vi "2 Round Buoy.vi"() -> ()   [LabVIEW 2011]
uses:
  2 Typedefs/UTM Location.ctl
  2 Typedefs/Velocity.ctl
  2 Classes/Mission/Mission.lvclass
  2 Globals/2 Global.vi
  2 Classes/MissionQueue/MissionQueue.lvclass
  2 Classes/Waypoint/Waypoint.lvclass
panel:
  in  "Tolerance":dbl=0.5
  out "First Waypoint":T1 {"North" format="%#_10f"; "East" format="%#_8f"}
  out "Third Waypoint":T1 {"North" format="%#_10f"; "East" format="%#_8f"}
  out "Second Waypoint":T1 {"North" format="%#_10f"; "East" format="%#_8f"}
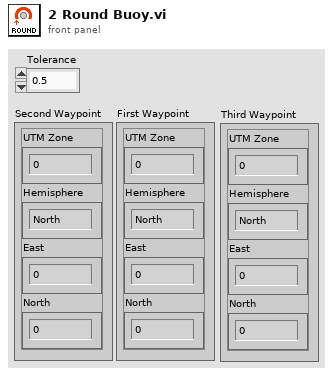
[diagram p1: front panel]
types:
  T1 = typedef "UTM Location.ctl" = cluster{"UTM Zone":dbl, "Hemisphere":enum16{"North", "South"}, "East":dbl, "North":dbl}
  T2 = typedef "Velocity.ctl" = cluster{"East":dbl, "North":dbl}
  T3 = cluster{"UTM Zone":dbl, "Hemisphere":u16, "East":dbl, "North":dbl}
  T4 = typedef "heading.ctl" = dbl
  T5 = typedef "Waypoints List.ctl" = refnum<class "Waypoint.lvclass">[]
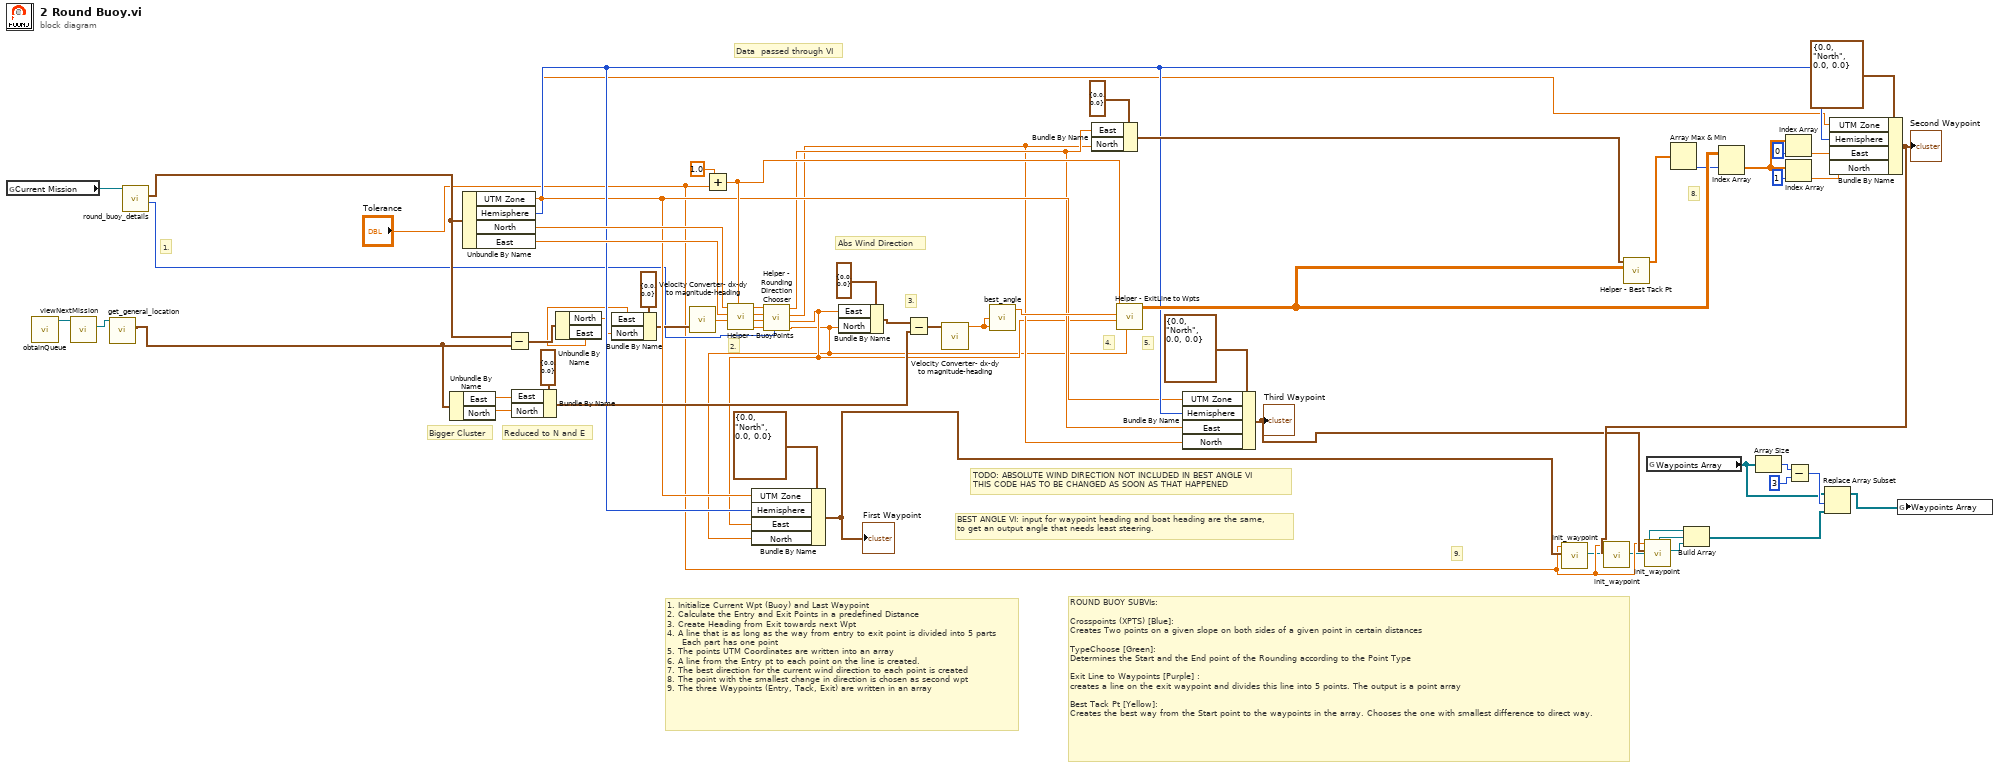
[diagram p0: block diagram]
diagram:
  # "ROUND BUOY SUBVIs:\n\nCrosspoints (XPTS) [Blue]:\nCreates Two points on a given slope on both sides of a given point in certain distances\n\nTypeChoose [Green]:\nDetermines the Start and the End point of the Rounding according to the Point Type\n\nExit Line to Waypoints [Purple] :\ncreates a line on the exit waypoint and divides this line into 5 points. The output is a point array\n\nBest Tack Pt [Yellow]:\nCreates the best way from the Start point to the waypoints in the array. Chooses the one with smallest difference to direct way."
  # "BEST ANGLE VI: input for waypoint heading and boat heading are the same,\nto get an output angle that needs least steering."
  # "Reduced to N and E"
  # "Bigger Cluster"
  # "Data  passed through VI"
  # "9."
  # "TODO: ABSOLUTE WIND DIRECTION NOT INCLUDED IN BEST ANGLE VI\nTHIS CODE HAS TO BE CHANGED AS SOON AS THAT HAPPENED"
  # "8."
  # "5."
  # "1. Initialize Current Wpt (Buoy) and Last Waypoint\n2. Calculate the Entry and Exit Points in a predefined Distance\n3. Create Heading from Exit towards next Wpt\n4. A line that is as long as the way from entry to exit point is divided into 5 parts\n     Each part has one point\n5. The points UTM Coordinates are written into an array\n6. A line from the Entry pt to each point on the line is created.\n7. The best direction for the current wind direction to each point is created\n8. The point with the smallest change in direction is chosen as second wpt\n9. The three Waypoints (Entry, Tack, Exit) are written in an array"
  # "4."
  # "3."
  # "Abs Wind Direction"
  # "2."
  # "1."
  n1 = global read "2 Global.vi" "Current Mission"() -> (w20:refnum<class "Mission.lvclass">)
  n2 = call "obtainQueue.vi"() -> ("MissionQueue.lvclass"=w17:refnum<class "MissionQueue.lvclass">)  [unwired: 10 in, 1 out]
  n3 = call "viewNextMission.vi"("MissionQueue in"=w17) -> ("Mission.lvclass"=w1:refnum<class "Mission.lvclass">)  [unwired: 7 in, 3 out]
  n4 = call "get_general_location.vi"("Mission in"=w1) -> ("General Location"=w2:T1)  [unwired: 8 in, 2 out]
  n5 = call-dynamic "round_buoy_details.vi"("Mission in"=w20) -> ("Round side?"=w18:enum16{"Starboard", "Port"}, "Buoy to Round"=w19:T1)  [unwired: 7 in, 2 out]
  n6 = Unbundle By Name(w2) -> ("East"=w58:dbl, "North"=w57:dbl)
  n7 = Unbundle By Name(w19) -> ("UTM Zone"=w35:dbl, "Hemisphere"=w36:enum16{"North", "South"}, "North"=w61:dbl, "East"=w60:dbl)
  n8 = Subtract(x=w19, y=w2) -> (x-y=w25:T3)
  n9 = Bundle By Name(cluster=T2 {"East"=0.0, "North"=0.0} ("Vector In"), "East"=w58, "North"=w57) -> (w54:T2)
  n10 = Unbundle By Name(w25) -> ("North"=w23:dbl, "East"=w16:dbl)
  n11 = Bundle By Name(cluster=T2 {"East"=0.0, "North"=0.0} ("Vector In"), "East"=w16, "North"=w23) -> (w22:T2)
  n12 = call "Velocity Converter- dx-dy to magnitude-heading.vi"("Vector In"=w22) -> ("Heading Out"=w21:T4)  [unwired: 9 in, 1 out]
  n13 = Add(x=1.0, y="Tolerance") -> (x+y=w52:dbl)
  n14 = call "Helper - BuoyPoints.vi"("Distance"=w52, "K"=w21, "East"=w60, "North"=w61) -> ("NorthOut 2"=w30:dbl, "East Out 2"=w31:dbl, "NorthOut"=w32:dbl, "East Out"=w33:dbl)  [unwired: 4 in]
  n15 = call "Helper - Rounding Direction Chooser.vi"("Enum"=w18, "Point NORTH 2"=w30, "Point EAST 2"=w31, "Point NORTH"=w32, "Point EAST"=w33) -> ("End Point NORTH"=w26:dbl, "End Point EAST"=w27:dbl, "Start Point NORTH"=w28:dbl, "Start Point EAST"=w29:dbl)  [unwired: 3 in]
  n16 = Bundle By Name(cluster=T1 {"UTM Zone"=0.0, "Hemisphere"=enum."North", "East"=0.0, "North"=0.0} ("UTM Location"), "UTM Zone"=w35, "Hemisphere"=w36, "East"=w27, "North"=w26) -> (w15:T1)
  "First Waypoint" <- w15
  n17 = Bundle By Name(cluster=T2 {"East"=0.0, "North"=0.0} ("Vector In"), "East"=w27, "North"=w26) -> (w40:T2)
  n18 = Subtract(x=w40, y=w54) -> (x-y=w53:T2)
  n19 = call "Velocity Converter- dx-dy to magnitude-heading.vi"("Vector In"=w53) -> ("Heading Out"=w34:T4)  [unwired: 9 in, 1 out]
  n20 = call "best_angle.vi"("Waypoint Heading"=w34, "Current Heading"=w34) -> ("Best Angle"=w51:dbl)  [unwired: 1 in, 2 out]
  n21 = Bundle By Name(cluster=T2 {"East"=0.0, "North"=0.0} ("Vector In"), "East"=w29, "North"=w28) -> (w41:T2)
  n22 = call "Helper - ExitLine to Wpts.vi"("NorthOut in"=w26, "East Out in"=w27, "Best Angle"=w51, "Dist/Time"=w52) -> ("Point on Line"=w48:dbl[][])  [unwired: 7 in]
  n23 = Bundle By Name(cluster=T1 {"UTM Zone"=0.0, "Hemisphere"=enum."North", "East"=0.0, "North"=0.0} ("UTM Location"), "UTM Zone"=w35, "Hemisphere"=w36, "East"=w29, "North"=w28) -> (w13:T1)
  "Third Waypoint" <- w13
  n24 = call "init_waypoint.vi"("Coords"=w15, "Tolerance (m)"="Tolerance") -> ("Waypoint Out"=w10:refnum<class "Waypoint.lvclass">)  [unwired: 9 in]
  n25 = call "Helper - Best Tack Pt.vi"("Point on Line"=w48, "Vector In"=w41) -> ("Array"=w49:dbl[])  [unwired: 9 in]
  n26 = call "init_waypoint.vi"("Coords"=w13, "Tolerance (m)"="Tolerance") -> ("Waypoint Out"=w8:refnum<class "Waypoint.lvclass">)  [unwired: 9 in]
  n27 = global read "2 Global.vi" "Waypoints Array"() -> (w5:T5)
  n28 = Array Max & Min(array=w49) -> (min index (indices)=w47:i32)  [unwired: 3 out]
  n29 = Index Array(array=w48, index (row)=w47) -> (element=w42:dbl[])  [unwired: 1 in]
  n30 = Array Size(array=w5) -> (size(s)=w11:i32)
  n31 = Index Array(array=w42, index=0) -> (element=w44:dbl)
  n32 = Index Array(array=w42, index=1) -> (element=w43:dbl)
  n33 = Subtract(x=w11, y=3) -> (x-y=w6:i32)
  n34 = Bundle By Name(cluster=T1 {"UTM Zone"=0.0, "Hemisphere"=enum."North", "East"=0.0, "North"=0.0} ("UTM Location"), "UTM Zone"=w35, "Hemisphere"=w36, "East"=w44, "North"=w43) -> (w14:T1)
  "Second Waypoint" <- w14
  n35 = call "init_waypoint.vi"("Coords"=w14, "Tolerance (m)"="Tolerance") -> ("Waypoint Out"=w9:refnum<class "Waypoint.lvclass">)  [unwired: 9 in]
  n36 = Build Array(w10, w9, w8) -> (w4:refnum<class "Waypoint.lvclass">[])
  n37 = Replace Array Subset(array=w5, new element=w4, index=w6) -> (w3:T5)
  n38 = global write "2 Global.vi" "Waypoints Array"(w3) -> ()
